vi "set agc mode.vi"(8 "error in (no error)":errorcluster, 10 "AGC Enable":bool, 11 "DeviceRefnum":u64) -> (0 "error out":errorcluster, 2 "function return":i32, 3 "DeviceRefnum Out":u64)   [LabVIEW 2015, in "rtlsdr.lvlib"]
doc: "Enable or disable the internal digital AGC of the RTL2832."
uses:
  rtlsdr.lvlib
  rtlsdr/rtlsdr.dll
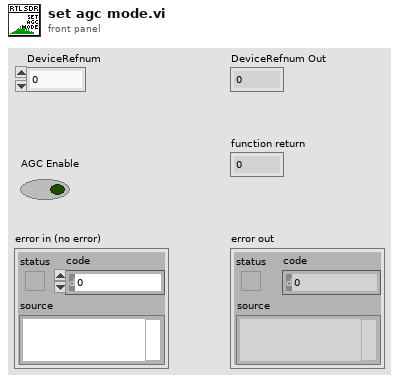
[diagram p1: front panel]
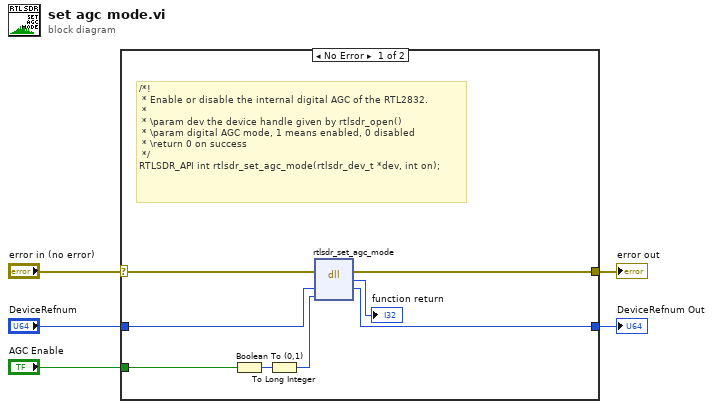
[diagram p0: block diagram]
diagram:
  n1 = case shown="No Error" "error in (no error)" {
    selector: "error in (no error)" -> [w6 w15]
    tunnel: [w12 w15] -> w5
    tunnel: "DeviceRefnum" -> [w11 w14]
    tunnel: [w10 w14] -> w3
    tunnel: "AGC Enable" -> [w9 _]
    frame No Error {
      # "/*!\n * Enable or disable the internal digital AGC of the RTL2832.\n *\n * \\param dev the device handle given by rtlsdr_open()\n * \\param digital AGC mode, 1 means enabled, 0 disabled\n * \\return 0 on success\n */\nRTLSDR_API int rtlsdr_set_agc_mode(rtlsdr_dev_t *dev, int on);"
      n2 = Boolean To (0,1)(Boolean=w9) -> (0, 1=w8:i16)
      n3 = To Long Integer(number=w8) -> (32bit integer=w7:i32)
      n4 = dll-call lib="C:/Users/TheDoctor/Documents/Projects/Labview Libraries/rtlsdr/rtlsdr.*" fn="rtlsdr_set_agc_mode"(error in=w6, "DeviceRefnum"=w11, "AGC Mode"=w7) -> (error out=w12:errorcluster, "return type"=→"function return":i32, "DeviceRefnum"=w10:u64)  [unwired: 3 in, 1 out]
    }
    frame Error {
    }
  }
  "error out" <- w5
  "DeviceRefnum Out" <- w3
